vi "Create File on Error.vi"(8 "error in (no error)":errorcluster, 11 "File Path":path) -> (0 "error out":errorcluster, 3 "File Path (dup)":path)   [LabVIEW 2019]
doc: "Create a file with the specified path if there is an error as input.\nReturns the path of the created file with no error if the file could be created (or replaced)."
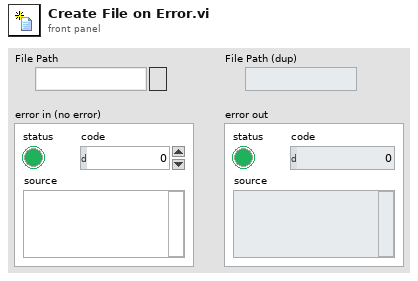
[diagram p1: front panel]
types:
  T1 = enum16{"open", "replace", "create", "open or create", "replace or create", "replace or create with confirmation"}
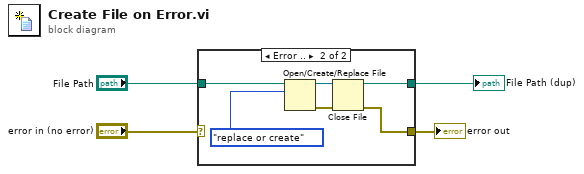
[diagram p0: block diagram]
diagram:
  n1 = case shown="Error .." "error in (no error)" {
    selector: "error in (no error)" -> [w5 _]
    tunnel: "File Path" -> [w6 w12]
    tunnel: [w6 w9] -> w2
    tunnel: [w5 w7] -> w1
    frame No Error {
    }
    frame Error {
      n2 = Open/Create/Replace File(file path (use dialog)=w12, operation (0:open)=T1."replace or create") -> (refnum out=w10:refnum<file>, error out=w8:errorcluster)  [unwired: 4 in, 1 out]
      n3 = Close File(refnum=w10, error in=w8) -> (path=w9:path, error out=w7:errorcluster)
    }
  }
  "error out" <- w1
  "File Path (dup)" <- w2
